vi "ring ioc motors.vi"(8 "error in":errorcluster) -> (0 "error out":errorcluster, 3 "Strings And Values Commands":cluster{"String":string, "Value":string}[](array[cluster]))   [LabVIEW 2022 SP3]
uses:
  pectus/global/global IOC database.vi
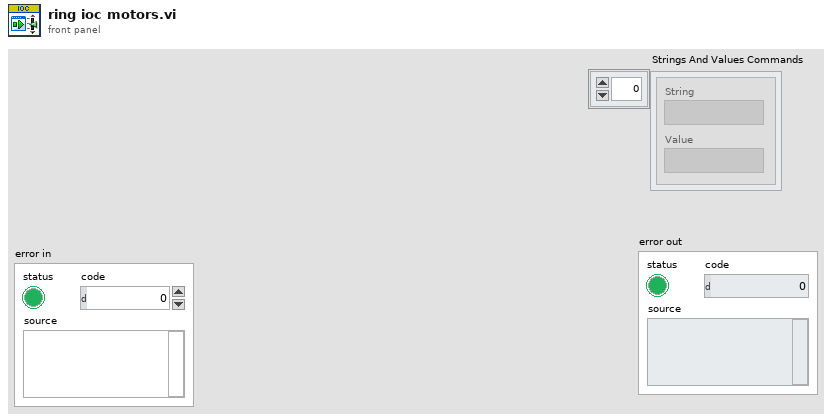
[diagram p1: front panel]
types:
  T1 = typedef "epics database.ctl" = cluster{"IOC":string, "db":string, "Field Values":string[], "Values":string[][], "Type":string, "Card":u16, "Num Dev":u16}
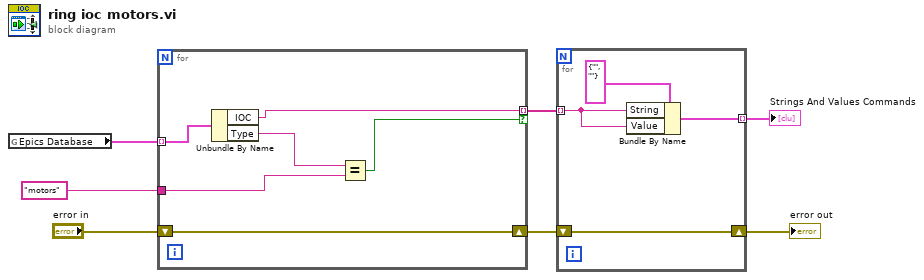
[diagram p0: block diagram]
diagram:
  n1 = global read "global IOC database.vi" "Epics Database"() -> (w7:T1[])
  n2 = for {
    tunnel: w7 -> [w13] mode=indexing
    tunnel: "motors" ("IOC") -> [w11]
    shift-right: [w10] -> w4
    shift-left: "error in" -> [w10]
    tunnel: [w9] -> w2 mode=indexing if=w8
    n3 = Unbundle By Name(w13) -> ("IOC"=w9:string, "Type"=w12:string)
    n4 = Equal?(x=w12, y=w11) -> (x = y?=w8:bool)
  }
  n5 = for {
    shift-right: [w17] -> w3
    shift-left: w4 -> [w17]
    tunnel: w2 -> [w15] mode=indexing
    tunnel: [w14] -> w1 mode=indexing
    n6 = Bundle By Name(cluster=cluster{"String":string, "Value":string} {"String"="", "Value"=""}, "String"=w15, "Value"=w15) -> (w14:cluster{"String":string, "Value":string})
  }
  "error out" <- w3
  "Strings And Values Commands" <- w1
